vi "Part 2.vi"(11 "Input":string) -> (3 "Output":i64)   [LabVIEW 2021]
uses:
  <userlib>/_OpenG.lib/string/string.llb/Convert EOLs (String)__ogtk.vi
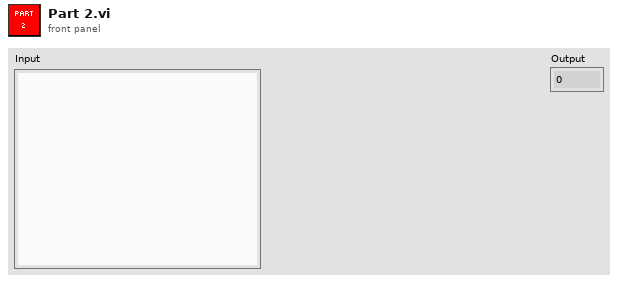
[diagram p1: front panel]
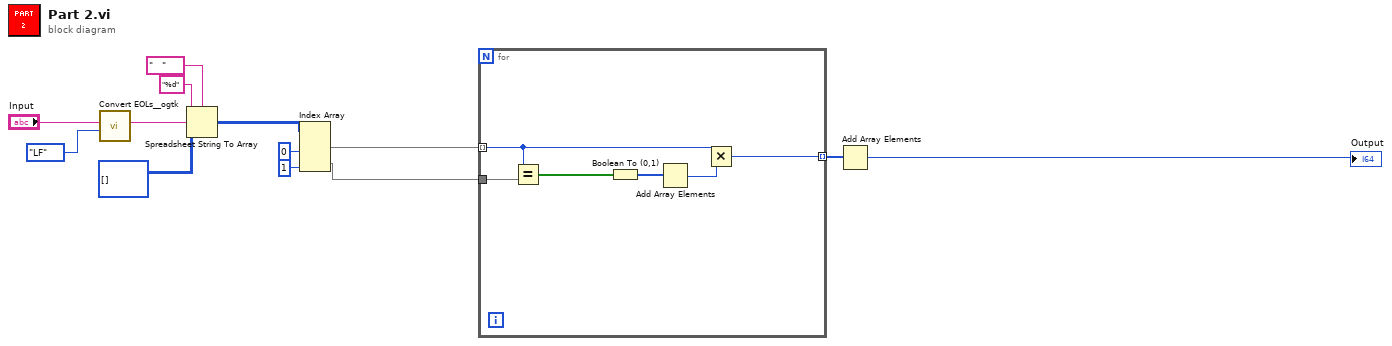
[diagram p0: block diagram]
diagram:
  n1 = call-poly <userlib>:"Convert EOLs__ogtk.vi"("Convert to:"=enum16{"CR", "LF", "CRLF"}."LF", "String in"="Input") -> ("String out"=w10:string)  [unwired: 9 in]
  n2 = Spreadsheet String To Array(delimiter (Tab)="   ", format string="%d", spreadsheet string=w10, array type (2D Dbl)=i64[][] []) -> (array=w8:i64[][])
  n3 = Index Array(array=w8, index (col) #1=0 ("disabled index (col)"), index (col) #2=1 ("index (col)")) -> (element #1=w4:i64[], element #2=w3:i64[])  [unwired: 2 in]
  n4 = for {
    tunnel: w4 -> [w16] mode=indexing
    tunnel: w3 -> [w19]
    tunnel: [w14] -> w2 mode=indexing
    n5 = Equal?(x=w16, y=w19) -> (x = y?=w18:bool[])
    n6 = Boolean To (0,1)(Boolean=w18) -> (0, 1=w17:i16[])
    n7 = Add Array Elements(numeric array=w17) -> (sum=w15:i16)
    n8 = Multiply(x=w16, y=w15) -> (x*y=w14:i64)
  }
  n9 = Add Array Elements(numeric array=w2) -> (sum=→"Output":i64)
